vi "Point_Create.vi"   [LabVIEW 2017, in "PointValueMap.lvlib"]
doc: "Creates a new map point with a specified name but without a value."
uses:
  <vilib>/addons/PointValueMap/PointValueMap.lvlib
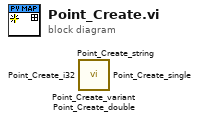
[diagram p0: block diagram]
diagram:
  n1 = call <vilib>:"Point_Create_variant.vi"() -> ()  [unwired: 10 in, 2 out]
  n2 = call <vilib>:"Point_Create_string.vi"() -> ()  [unwired: 10 in, 2 out]
  n3 = call <vilib>:"Point_Create_i32.vi"() -> ()  [unwired: 10 in, 2 out]
  n4 = call <vilib>:"Point_Create_single.vi"() -> ()  [unwired: 10 in, 2 out]
  n5 = call <vilib>:"Point_Create_double.vi"() -> ()  [unwired: 10 in, 2 out]
